vi "FTW-ActorRef-SpawnNewActor.vi"(0 "Actor Ref Prototype":refnum<class "FTW-ActorReference.lvclass">, 11 "error in":errorcluster) -> (4 "Actor Reference":refnum<class "FTW-ActorReference.lvclass">, 15 "error out":errorcluster)   [LabVIEW 2013, in "FTW-ActorReference.lvclass"]
uses:
  FTW-ActorReference.lvclass
  FTW-ActorReference.lvclass/FTW-ActorReference.ctl
  Context/FTW-Actor-Context.lvclass
  Messaging/Address/FTW-Actor-Address.lvclass
panel:
  # "Inputs"
  # "Outputs"
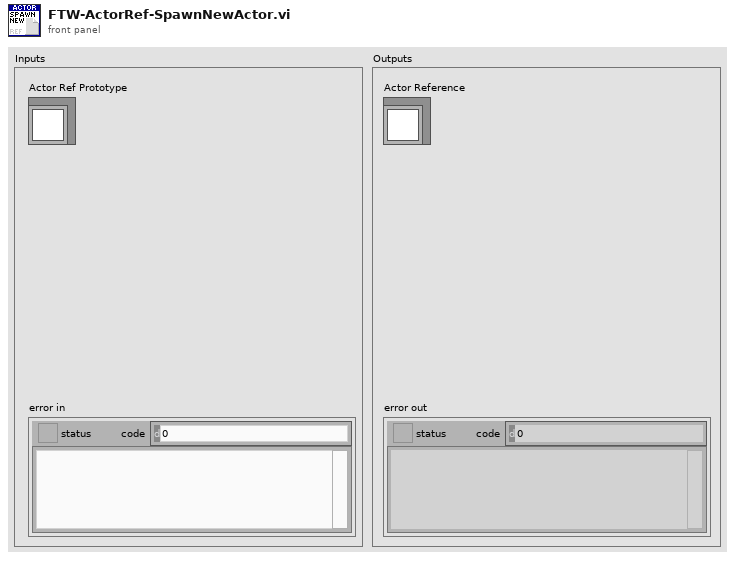
[diagram p1: front panel]
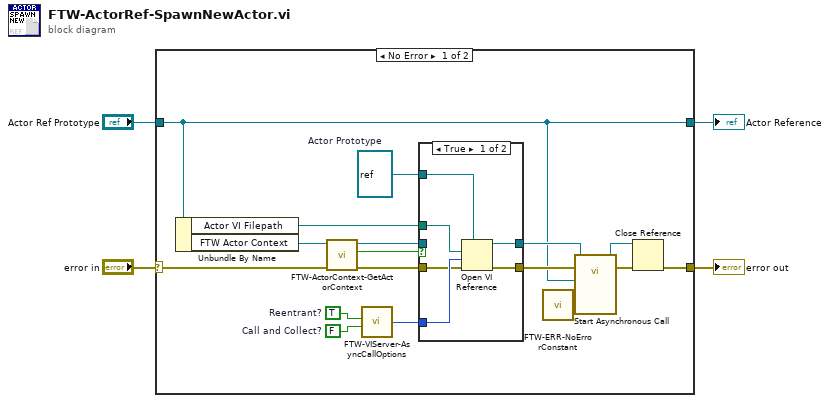
[diagram p0: block diagram]
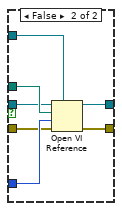
[diagram p2: hidden frame]
diagram:
  n1 = case shown="No Error" "error in" {
    selector: "error in" -> [w6 w36]
    tunnel: "Actor Ref Prototype" -> [w13 w35]
    tunnel: [w13 w35] -> w4
    tunnel: [w12 w36] -> w3
    frame No Error {
      w10 = refnum<vi> refnum  # Actor Prototype
      w18 = FALSE  # Call and Collect?
      w19 = TRUE  # Reentrant?
      n2 = Unbundle By Name(w13) -> ("Actor VI Filepath"=w11:path, "FTW Actor Context"=w9:refnum<class "FTW-Actor-Context.lvclass">)
      n3 = call "FTW-ActorContext-GetActorContext.vi"("error in"=w6, "Actor Context"=w9) -> ("error out"=w5:errorcluster, "Use Local Context"=w8:bool, "Actor Context"=w7:refnum<vi>)  [unwired: 7 in]
      n4 = call "FTW-VIServer-AsyncCallOptions.vi"("Call and Collect?"=w18, "Reentrant?"=w19) -> ("Open VI Ref Options"=w20:i32)  [unwired: 4 in]
      n5 = case shown="True" w8 {
        tunnel: [w27 w34] -> w21
        tunnel: w20 -> [w26 w33]
        tunnel: [w25 w32] -> w17
        tunnel: w7 -> [_ w28]
        tunnel: w5 -> [w24 w31]
        tunnel: w10 -> [w23 w30]
        tunnel: w11 -> [w22 w29]
        frame True {
          n6 = Open VI Reference(type specifier VI Refnum (for type only)=w23, vi path=w22, options=w26, error in (no error)=w24) -> (vi reference=w25:refnum<vi>, error out=w27:errorcluster)  [unwired: 2 in]
        }
        frame False {
          n7 = Open VI Reference(type specifier VI Refnum (for type only)=w30, application reference (local)=w28, vi path=w29, options=w33, error in (no error)=w31) -> (vi reference=w32:refnum<vi>, error out=w34:errorcluster)  [unwired: 1 in]
        }
      }
      n8 = call "FTW-ERR-NoErrorConstant.vi"() -> ("no error"=w14:errorcluster)
      n9 = call-by-ref "Start Asynchronous Call"(reference=w17, error in=w21, "Actor Ref Prototype"=w13, "error in"=w14) -> (reference out=w15:refnum<vi>, error out=w16:errorcluster)  [unwired: 13 in, 1 out]
      n10 = Close Reference(reference=w15, error in (no error)=w16) -> (error out=w12:errorcluster)
    }
    frame Error {
    }
  }
  "error out" <- w3
  "Actor Reference" <- w4
